vi "Read Port.vi"(0 "Serial Device in":refnum<class "Serial Device.lvclass">, 5 "VISA resource name":refnum<visa-resource-name>, 7 "Port":dbl, 11 "error in (no error)":errorcluster) -> (4 "Serial Device out":refnum<class "Serial Device.lvclass">, 6 "VISA resource name 2":refnum<visa-resource-name>, 8 "Binary Number":T1, 10 "Response":string, 15 "error out":errorcluster)   [LabVIEW 2020, in "Serial Device.lvclass"]
uses:
  Serial Device.lvclass
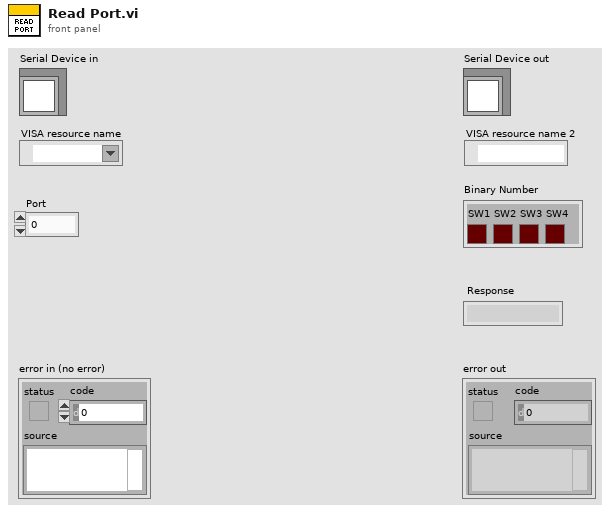
[diagram p1: front panel]
types:
  T1 = cluster{"SW1":bool, "SW2":bool, "SW3":bool, "SW4":bool}
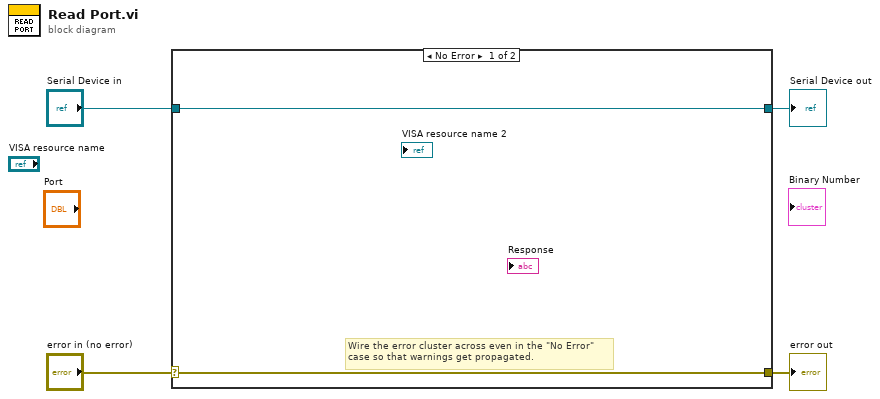
[diagram p0: block diagram]
diagram:
  n1 = case shown="No Error" "error in (no error)" {
    selector: "error in (no error)" -> [w5 w8]
    tunnel: [w5 w8] -> w3
    tunnel: [w6 w7] -> w1
    tunnel: "Serial Device in" -> [w6 w7]
    frame No Error {
      # "Wire the error cluster across even in the \"No Error\"\ncase so that warnings get propagated."
    }
    frame Error {
    }
  }
  "error out" <- w3
  "Serial Device out" <- w1
